vi "FRCts20_Backend_Error_Handler.vi"(6 "Failed Message":T4, 8 "Error In":errorcluster, 11 "Engine_Refnums In":T1) -> (0 "error out":errorcluster, 3 "Engine_Refnums Out":T1)   [LabVIEW 2013, in "FRCts20_Backend_Engine.lvlib"]
uses:
  FRCts20_Backend_Engine.lvlib
  FRCts20_Backend_EngineRefnums.ctl
  INI_Accessor/FRCts20_Backend_INI Controller.lvclass
  Dependencies/AMC/_SubVIs/TypeDefs/Message Queue.ctl
  Dependencies/AMC/_SubVIs/TypeDefs/Message.ctl
  Dependencies/Keyed Array/KeyedArray.ctl
  <vilib>/addons/database/Connection.llb/Conn ObjectReference.ctl
  FRCts20_Backend_FGVOperation.ctl
  Dependencies/Keyed Array/Tools_KeyedArray.lvlib
  Dependencies/AMC/AMC.lvlib
  <vilib>/addons/database/NI_Database_API.lvlib
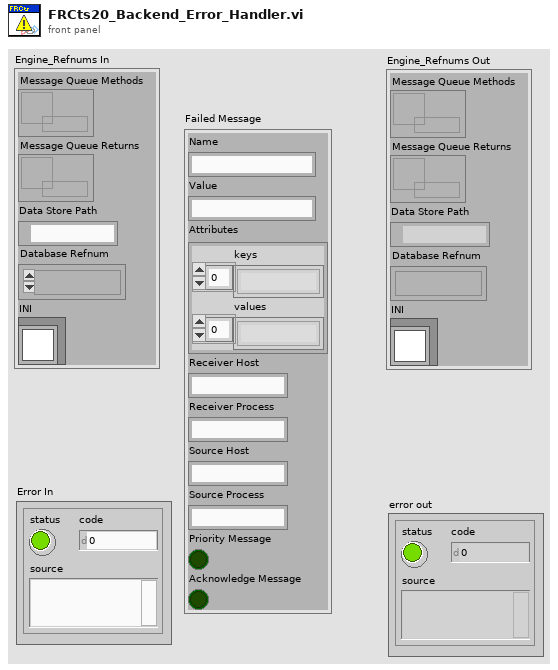
[diagram p1: front panel]
types:
  T1 = typedef "FRCts20_Backend_Engine.lvlib/FRCts20_Backend_EngineRefnums.ctl" = cluster{"Message Queue Methods":T2, "Message Queue Returns":T2, "Data Store Path":path, "Database Refnum":T3, "INI":refnum<class "FRCts20_Backend_INI Controller.lvclass">}
  T2 = typedef "AMC.lvlib/Message Queue.ctl" = refnum<queue>
  T3 = typedef "NI_Database_API.lvlib/Conn ObjectReference.ctl" = refnum<k1>
  T4 = typedef "AMC.lvlib/Message.ctl" = cluster{"Name":string, "Value":string, "Attributes":T5, "Receiver Host":string, "Receiver Process":string, "Source Host":string, "Source Process":string, "Priority Message":bool, "Acknowledge Message":bool}
  T5 = typedef "Tools_KeyedArray.lvlib/KeyedArray.ctl" = cluster{"keys":string[], "values":string[]}
  T6 = typedef "FRCts20_Backend_Engine.lvlib/FRCts20_Backend_FGVOperation.ctl" = enum16{"Initialize", "EnqueueMessage", "EnqueueDataReturn", "FlushMessage", "FlushDataReturn"}
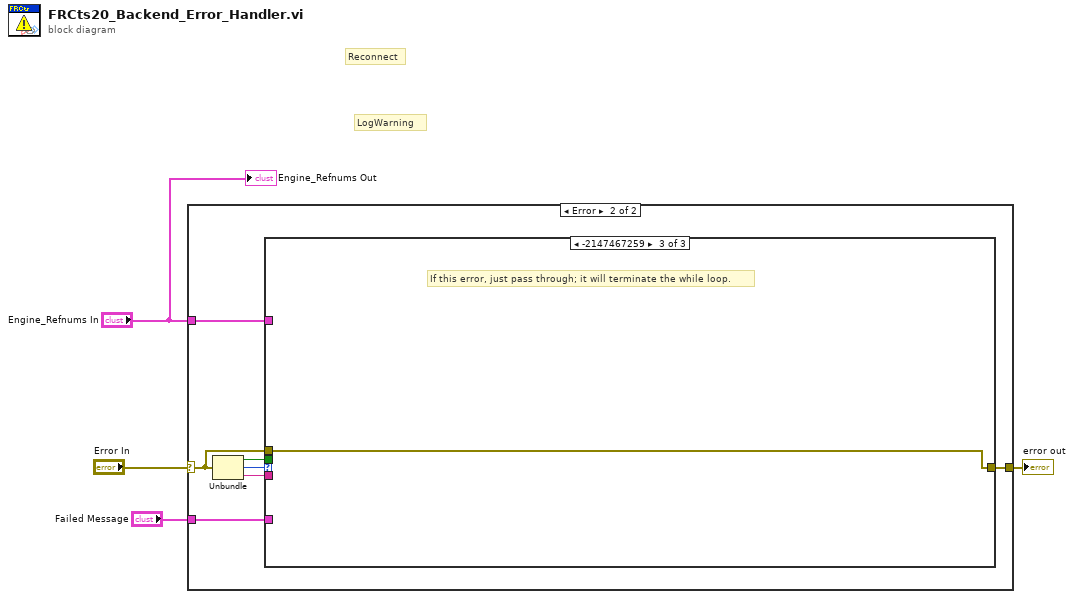
[diagram p0: block diagram]
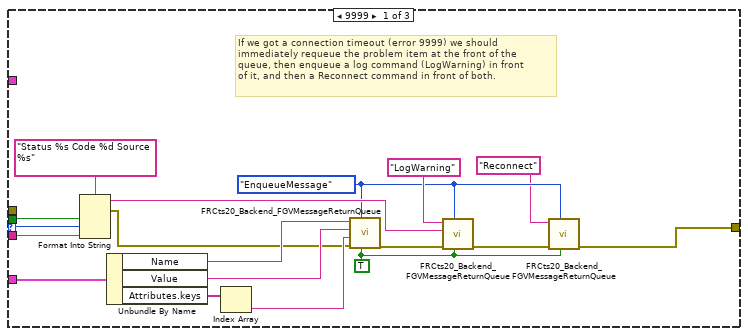
[diagram p3: hidden frame]
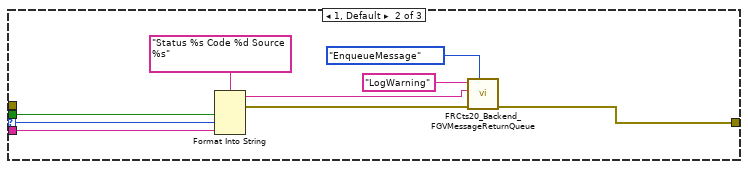
[diagram p4: hidden frame]
diagram:
  # "LogWarning"
  # "Reconnect"
  n1 = case shown="Error" "Error In" {
    selector: "Error In" -> [w5 w6]
    tunnel: [w5 w7] -> w3
    tunnel: "Engine_Refnums In" -> [_ w9]
    tunnel: "Failed Message" -> [_ w8]
    frame No Error {
    }
    frame Error {
      n2 = Unbundle(w6) -> ("status"=w11:bool, "code"=w10:i32, "source"=w12:string)
      n3 = case shown="-2147467259" w10 {
        selector: w10 -> [w22 w32 _]
        tunnel: w12 -> [w21 w31 _]
        tunnel: w11 -> [w23 w33 _]
        tunnel: w9 -> [_ _ _]
        tunnel: w8 -> [w30 _ _]
        tunnel: [w13 w34 w40] -> w7
        tunnel: w6 -> [_ _ w40]
        frame 9999 {
          w16 = TRUE ("Priority Message (F)")
          w15 = FRCts20_Backend_FGVOperation."EnqueueMessage" ("Operation")
          # "If we got a connection timeout (error 9999) we should\nimmediately requeue the problem item at the front of the\nqueue, then enqueue a log command (LogWarning) in front\nof it, and then a Reconnect command in front of both."
          n4 = Format Into String(format string="Status %s Code %d Source %s", w23, w22, w21) -> (resulting string=w18:string, error out=w19:errorcluster)  [unwired: 2 in]
          n5 = Unbundle By Name(w30) -> ("Name"=w27:string, "Value"=w26:string, "Attributes.keys"=w29:string[])
          n6 = Index Array(array=w29) -> (element=w28:string)  [unwired: 1 in]
          n7 = call "FRCts20_Backend_FGVMessageReturnQueue.vi"("Priority Message (F)"=w16, "Operation"=w15, "error in (no error)"=w19, "Key"=w28, "Message Value"=w26, "Message Name"=w27) -> ("error out"=w25:errorcluster)  [unwired: 4 in, 1 out]
          n8 = call "FRCts20_Backend_FGVMessageReturnQueue.vi"("Priority Message (F)"=w16, "Operation"=w15, "error in (no error)"=w25, "Message Value"=w18, "Message Name"="LogWarning") -> ("error out"=w17:errorcluster)  [unwired: 5 in, 1 out]
          n9 = call "FRCts20_Backend_FGVMessageReturnQueue.vi"("Priority Message (F)"=w16, "Operation"=w15, "error in (no error)"=w17, "Message Name"="Reconnect") -> ("error out"=w13:errorcluster)  [unwired: 6 in, 1 out]
        }
        frame 1, Default {
          n10 = Format Into String(format string="Status %s Code %d Source %s", w33, w32, w31) -> (resulting string=w35:string, error out=w36:errorcluster)  [unwired: 2 in]
          n11 = call "FRCts20_Backend_FGVMessageReturnQueue.vi"("Operation"=FRCts20_Backend_FGVOperation."EnqueueMessage", "error in (no error)"=w36, "Message Value"=w35, "Message Name"="LogWarning") -> ("error out"=w34:errorcluster)  [unwired: 6 in, 1 out]
        }
        frame -2147467259 {
          # "If this error, just pass through; it will terminate the while loop."
        }
      }
    }
  }
  "error out" <- w3
  "Engine_Refnums Out" <- "Engine_Refnums In"
